vi "Launching Static VI.vi"(9 "Data To Set":T1[](array[typedef]), 11 "VI Ref In":refnum<vi>) -> ()   [LabVIEW 2019]
uses:
  TypeDef/Static VI Launch Input.ctl
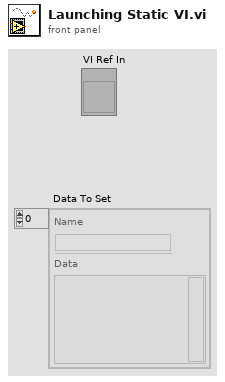
[diagram p1: front panel]
types:
  T1 = typedef "Static VI Launch Input.ctl" = cluster{"Name":string, "Data":variant}
  T2 = enum32{"Bad", "Idle", "Run top level", "Running"}
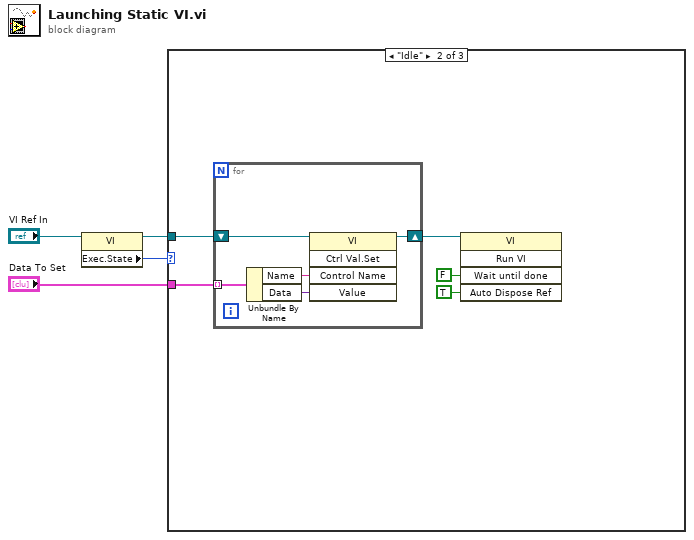
[diagram p0: block diagram]
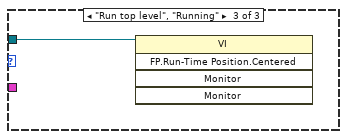
[diagram p3: hidden frame]
diagram:
  n1 = property class="VI"(reference="VI Ref In") -> (reference out=w2:refnum<vi>, "Exec.State"=w3:T2)  [unwired: 1 in, 1 out]
  n2 = case shown="\"Idle\"" w3 {
    tunnel: w2 -> [_ w9 w15]
    tunnel: "Data To Set" -> [_ w8 _]
    frame "Bad", Default {
    }
    frame "Idle" {
      n3 = for {
        tunnel: w8 -> [w13] mode=indexing
        shift-right: [w10] -> w7
        shift-left: w9 -> [w14]
        n4 = Unbundle By Name(w13) -> ("Name"=w12:string, "Data"=w11:variant)
        n5 = invoke class="VI" method="Ctrl Val.Set"(reference=w14, "Control Name"=w12, "Value"=w11) -> (reference out=w10:refnum<vi>)  [unwired: 2 in, 4 out]
      }
      n6 = invoke class="VI" method="Run VI"(reference=w7, "Wait until done"=FALSE ("Wait Until Done"), "Auto Dispose Ref"=TRUE ("Auto Dispose Reference")) -> ()  [unwired: 2 in, 5 out]
    }
    frame "Run top level", "Running" {
      n7 = invoke class="VI" method="FP.Run-Time Position.Centered"(reference=w15) -> ()  [unwired: 4 in, 5 out]
    }
  }
